vi "Delay Graph inquiry.vi"(0 "VISA resource name":refnum<visa-resource-name>, 1 "Number":dbl, 3 "Count":dbl, 5 "Channel  (1: CH1)":u16(ring)=1 items=["CH1"=1, "CH2"=2, "CH3"=3, "CH4"=4], 11 "error in (no error)":errorcluster, 12 "Calculate":bool, 14 "Plot":bool) -> (4 "VISA resource name out":refnum<visa-resource-name>, 6 "Graph":dynamicdata(graph), 8 "Table":string[][](table), 15 "error out":errorcluster)   [LabVIEW 2020, in "GPP.lvlib"]
uses:
  GPP.lvlib
  <vilib>/Platform/TimedLoop/XDataNode/timing_clust.ctl
  <vilib>/Platform/TimedLoop/XDataNode/nitl_modes.ctl
  <vilib>/Platform/TimedLoop/XDataNode/wakeup.ctl
  Function/VISA_COMMON.ctl
  <vilib>/Platform/TimedLoop/XDataNode/XDataNode.xnode
  <vilib>/Platform/TimedLoop/XDataNode/XDNodeRunTimeDep.lvlib
panel:
  out "ON/OFF 2":dbl[](array[numeric])
  in  "历史数据":dynamicdata[](array[waveform])
  in  "Table 4":string[][](table)
  in  "历史数据 2":dynamicdata[](array[waveform])
  in  "Table 5":string[][](table)
  in  "In":string
  out "CUT HEAD":string
  out "ADD ;":string
  out "CUT ;":string
  out "AFTER CUT":string
  out "CUT LAST":string
  out "Time 2":dbl
  out "Time 3":dbl
  out "Number 3":dbl
  out "ON/OFF":string[](array[string])
  out "Time":dbl[](array[numeric])
  out "Number 2":dbl[](array[numeric])
  out "on/off":string
  out "Stay":string
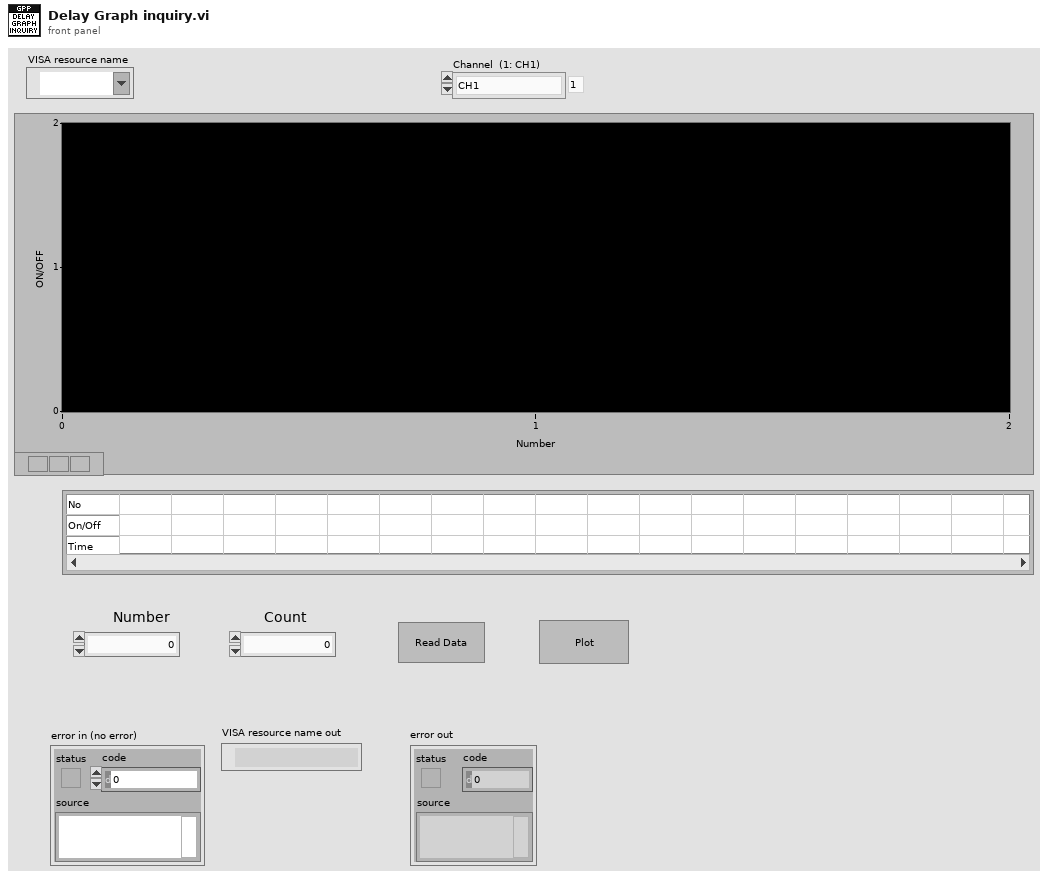
[diagram p1: front panel]
types:
  T1 = typedef "XDNodeRunTimeDep.lvlib/timing_clust.ctl" = cluster{"Expected End [f-1]":u64, "Actual End [f-1]":u64, "Finished Late? [f-1]":bool, "Expected End [i-1]":u64, "Actual End [i-1]":u64, "Finished Late? [i-1]":bool, "Expected Start [i]":u64, "Actual Start [i]":u64, "Expected Start [f]":u64, "Actual Start [f]":u64, "Source Name":string, "Structure Name":string, "Period":i64, "Deadline":i64, "Offset":i64, "Start":i64, "Priority":i32, "Timeout":i32, "Mode":T2, "Wakeup Reason":T3, "Error":errorcluster, "Source Type":string, "Secondary Source Type":string, "Global End Time":u64, "Global Start Time":u64, "Frame Duration":u64, "Iteration Duration":u64, "Assigned CPU":i32, "I/O Scan Engine Mode":u32}
  T2 = typedef "XDNodeRunTimeDep.lvlib/nitl_modes.ctl" = enum32{"No Change", "Process missed periods, maintain original phase", "Discard missed periods, maintain original phase", "Process missed periods, ignore original phase", "Discard missed periods, ignore original phase"}
  T3 = typedef "XDNodeRunTimeDep.lvlib/wakeup.ctl" = enum32{"Normal", "Aborted", "Asynchronous wakeup", "Timing source error", "Timed loop error", "Timeout"}
  T4 = typedef "GPP.lvlib/VISA_COMMON.ctl" = enum16{"Initial", "Write CMD", "Read Result", "Read History", "Close"}
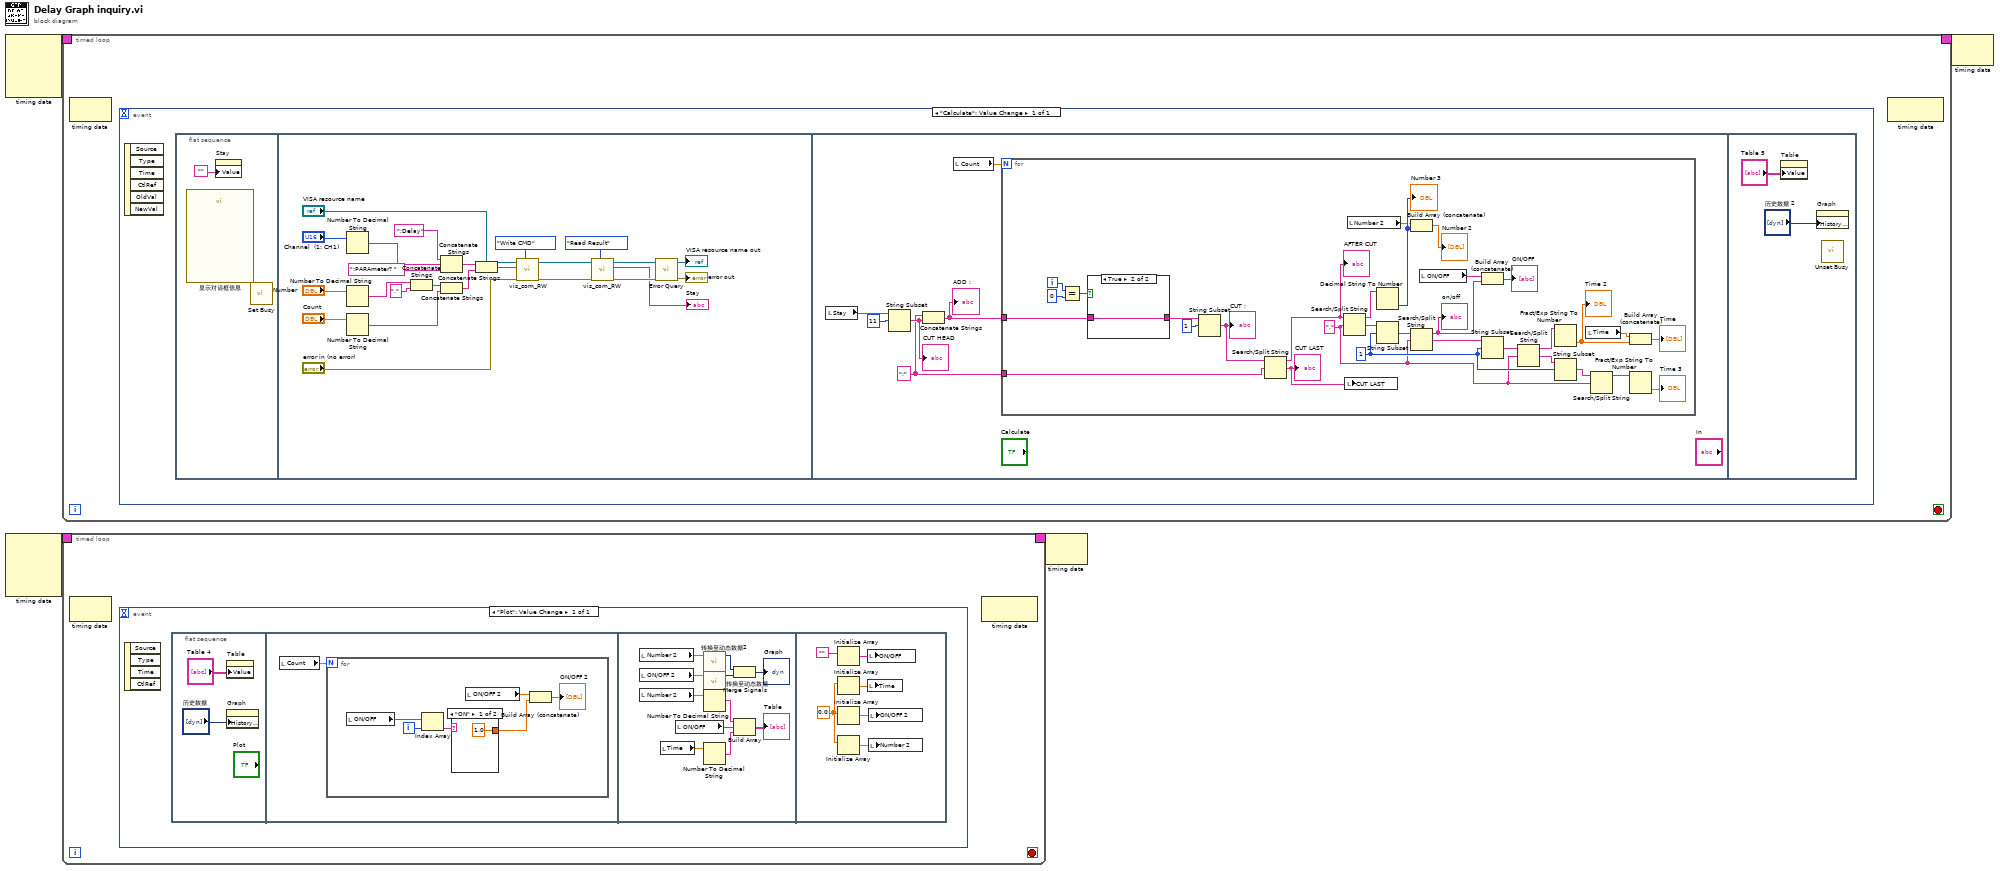
[diagram p0: block diagram]
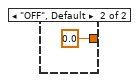
[diagram p2: hidden frame]
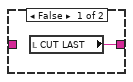
[diagram p3: hidden frame]
diagram:
  n1 = node-c288() -> (w4:T1)  [unwired: 4 in]
  n2 = node-c288() -> (w2:T1)  [unwired: 4 in]
  n3 = timed-loop {
    timing: w4 -> [_]
    timing-out: [_] -> w3
    stop <- _ stop-if-true
    n4 = node-c288() -> ()  [unwired: 1 in, 1 out]
    n5 = event shown="[0] \"Calculate\": Value Change" {
      selector: _ -> [_]
      dyn-events: _ -> [_]
      timeout: _ -> [_]
      event "Calculate": Value Change {
        n6 = event-data() -> ()  [unwired: 1 in, 6 out]
        n7 = flat-sequence {
          frame #0 {
            n8 = call "显示对话框信息"() -> ()  [unwired: 10 in, 2 out]
            n9 = property on="Stay" class="Str"("Value"="") -> ()  [unwired: 2 in, 2 out]
            n10 = call <vilib>:"Set Busy.vi"() -> ()  [unwired: 10 in, 2 out]
          }
          frame #1 {
            n11 = Number To Decimal String(number="Channel  (1: CH1)") -> (decimal integer string=w19:string)  [unwired: 1 in]
            n12 = Number To Decimal String(number="Number") -> (decimal integer string=w29:string)  [unwired: 1 in]
            n13 = Number To Decimal String(number="Count") -> (decimal integer string=w26:string)  [unwired: 1 in]
            n14 = Concatenate Strings(w29, ",") -> (w27:string)
            n15 = Concatenate Strings(":Delay", w19, ":PARAmeter? ") -> (w17:string)
            n16 = Concatenate Strings(w27, w26) -> (w25:string)
            n17 = Concatenate Strings(w17, w25) -> (w24:string)
            n18 = call "vis_com_RW.vi"("Funciton"=VISA_COMMON."Write CMD", "error in (no error)"="error in (no error)", "CMD String"=w24, "VISA resource in"="VISA resource name") -> ("error out"=w12:errorcluster, "VISA resource out"=w9:refnum<visa-resource-name>)  [unwired: 5 in, 1 out]
            n19 = call "vis_com_RW.vi"("Funciton"=VISA_COMMON."Read Result", "error in (no error)"=w12, "VISA resource in"=w9) -> ("error out"=w10:errorcluster, "Result"=→"Stay":string, "VISA resource out"=w8:refnum<visa-resource-name>)  [unwired: 6 in]
            n20 = call "Error Query.vi"("error in (no error)"=w10, "VISA resource name"=w8) -> ("error out"=→"error out":errorcluster, "VISA resource name out"=→"VISA resource name out":refnum<visa-resource-name>)  [unwired: 6 in, 2 out]
          }
          frame #2 {
            w33 = ";"
            n21 = local read "Stay"() -> (w30:string)
            n22 = String Subset(string=w30, offset (0)=11) -> (substring=w34:string)  [unwired: 1 in]
            "CUT HEAD" <- w34
            n23 = Concatenate Strings(w33, w34) -> (w32:string)
            "ADD ;" <- w32
            n24 = local read "Count"() -> (w31:dbl)
            n25 = for {
              N: w31 -> [_]
              tunnel: w33 -> [w66]
              tunnel: w32 -> [w38]
              i -> [w40]
              w56 = 1
              w54 = ","
              n26 = Equal?(x=w40, y=0) -> (x = y?=w39:bool)
              n27 = case shown="True" w39 {
                tunnel: w38 -> [_ w68]
                tunnel: [w67 w68] -> w37
                frame False {
                  n28 = local read "CUT LAST"() -> (w67:string)
                }
                frame True {
                }
              }
              n29 = String Subset(string=w37, offset (0)=1) -> (substring=w65:string)  [unwired: 1 in]
              "CUT ;" <- w65
              n30 = Search/Split String(string=w65, search string/char (-)=w66) -> (substring before match=w62:string, match + rest of string=w63:string)  [unwired: 1 in, 1 out]
              "AFTER CUT" <- w62
              "CUT LAST" <- w63
              n31 = Search/Split String(string=w62, search string/char (-)=w54) -> (substring before match=w51:string, match + rest of string=w61:string)  [unwired: 1 in, 1 out]
              n32 = local write "CUT LAST"(w63) -> ()
              n33 = local read "Number 2"() -> (w44:dbl[])
              n34 = Decimal String To Number(string=w51) -> (number=w45:i32)  [unwired: 2 in, 1 out]
              "Number 3" <- w45
              n35 = String Subset(string=w61, offset (0)=w56) -> (substring=w60:string)  [unwired: 1 in]
              n36 = Build Array (concatenate)(w44, w45) -> (→"Number 2":dbl[])
              n37 = Search/Split String(string=w60, search string/char (-)=w54) -> (substring before match=w36:string, match + rest of string=w59:string)  [unwired: 1 in, 1 out]
              "on/off" <- w36
              n38 = local read "ON/OFF"() -> (w47:string[])
              n39 = Build Array (concatenate)(w47, w36) -> (→"ON/OFF":string[])
              n40 = String Subset(string=w59, offset (0)=w56) -> (substring=w58:string)  [unwired: 1 in]
              n41 = Search/Split String(string=w58, search string/char (-)=w54) -> (substring before match=w53:string, match + rest of string=w57:string)  [unwired: 1 in, 1 out]
              n42 = Fract/Exp String To Number(string=w53) -> (number=w49:dbl)  [unwired: 3 in, 1 out]
              "Time 2" <- w49
              n43 = String Subset(string=w57, offset (0)=w56) -> (substring=w55:string)  [unwired: 1 in]
              n44 = local read "Time"() -> (w46:dbl[])
              n45 = Search/Split String(string=w55, search string/char (-)=w54) -> (substring before match=w52:string)  [unwired: 1 in, 2 out]
              n46 = Build Array (concatenate)(w46, w49) -> (→"Time":dbl[])
              n47 = Fract/Exp String To Number(string=w52) -> (number=→"Time 3":dbl)  [unwired: 3 in, 1 out]
            }
          }
          frame #3 {
            n48 = property on="Table" class="Tbl (strict)"("Value"="Table 5") -> ()  [unwired: 2 in, 2 out]
            n49 = property on="Graph" class="WFChart (strict)"("History Data"="历史数据 2") -> ()  [unwired: 2 in, 2 out]
            n50 = call <vilib>:"Unset Busy.vi"() -> ()  [unwired: 11 in, 1 out]
          }
        }
      }
    }
    n51 = node-c288() -> ()  [unwired: 1 in, 1 out]
  }
  n52 = timed-loop {
    timing: w2 -> [_]
    timing-out: [_] -> w1
    stop <- _ stop-if-true
    n53 = node-c288() -> ()  [unwired: 1 in, 1 out]
    n54 = event shown="[0] \"Plot\": Value Change" {
      selector: _ -> [_]
      dyn-events: _ -> [_]
      timeout: _ -> [_]
      event "Plot": Value Change {
        n55 = event-data() -> ()  [unwired: 1 in, 4 out]
        n56 = flat-sequence {
          frame #0 {
            n57 = property on="Table" class="Tbl (strict)"("Value"="Table 4") -> ()  [unwired: 2 in, 2 out]
            n58 = property on="Graph" class="WFChart (strict)"("History Data"="历史数据") -> ()  [unwired: 2 in, 2 out]
          }
          frame #1 {
            n59 = local read "Count"() -> (w75:dbl)
            n60 = for {
              N: w75 -> [_]
              i -> [w81]
              n61 = local read "ON/OFF"() -> (w80:string[])
              n62 = Index Array(array=w80, index=w81) -> (element=w79:string)
              n63 = case shown="\"ON\"" w79 {
                tunnel: [1.0 0.0] -> w78
                frame "ON" {
                }
                frame "OFF", Default {
                }
              }
              n64 = local read "ON/OFF 2"() -> (w76:dbl[])
              n65 = Build Array (concatenate)(w76, w78) -> (→"ON/OFF 2":dbl[])
            }
          }
          frame #2 {
            n66 = local read "Number 2"() -> (w94:dbl[])
            n67 = local read "ON/OFF 2"() -> (w86:dbl[])
            n68 = local read "Number 2"() -> (w88:dbl[])
            n69 = local read "Time"() -> (w84:dbl[])
            n70 = local read "ON/OFF"() -> (w87:string[])
            n71 = call "转换至动态数据2"("Array"=w94) -> ("Dynamic Data Type"=w93:dynamicdata)  [unwired: 3 in]
            n72 = call "转换至动态数据"("Array"=w86) -> ("Dynamic Data Type"=w92:dynamicdata)  [unwired: 3 in]
            n73 = Number To Decimal String(number=w88) -> (decimal integer string=w89:string[])  [unwired: 1 in]
            n74 = Number To Decimal String(number=w84) -> (decimal integer string=w85:string[])  [unwired: 1 in]
            n75 = Merge Signals(w93, w92) -> (→"Graph":dynamicdata)
            n76 = Build Array(w89, w87, w85) -> (→"Table":string[][])
          }
          frame #3 {
            w95 = 0.0
            n77 = Initialize Array("") -> (w98:string[])  [unwired: 1 in]
            n78 = Initialize Array(w95) -> (w99:dbl[])  [unwired: 1 in]
            n79 = Initialize Array(w95) -> (w96:dbl[])  [unwired: 1 in]
            n80 = Initialize Array(w95) -> (w100:dbl[])  [unwired: 1 in]
            n81 = local write "ON/OFF"(w98) -> ()
            n82 = local write "Time"(w99) -> ()
            n83 = local write "ON/OFF 2"(w96) -> ()
            n84 = local write "Number 2"(w100) -> ()
          }
        }
      }
    }
    n85 = node-c288() -> ()  [unwired: 1 in, 1 out]
  }
  n86 = node-c288(w1) -> ()  [unwired: 1 out]
  n87 = node-c288(w3) -> ()  [unwired: 1 out]
